vi "initialize.vi"(0 "MoAgSy_Engine":refnum<class "MoAgSy_Engine.lvclass">, 3 "initializationData":variant, 5 "error in (no error)":errorcluster, 7 "binaryString":string, 8 "I8 Array":i8[](array[numeric]), 9 "prependSize? (T)":bool, 11 "byteOrder (0:big-endian, network order)":T1(ring)) -> (14 "dup MoAgSy_Engine":refnum<class "MoAgSy_Engine.lvclass">, 17 "found?":bool, 19 "error out":errorcluster)   [LabVIEW 2009, in "MoAgSy.lvlib" / "MoAgSy_Engine.lvclass"]
doc: "This is a dynamic dispatch VI to be implemented by child classes to initialize their attributes.\n\n<B>Recommendation:</B> Use Variant for initialization data."
uses:
  MoAgSy_Engine.lvclass
  MoAgSy_AgentBase/MoAgSy_AgentBase.lvclass
  HGF_BaseClasses/HGF_Event/HGF_Event.lvclass
  HGF_BaseClasses/HGF_ThreadTask/HGF_ThreadTask.lvclass
  MoAgSy_Engine.lvclass/MoAgSy_Engine.ctl
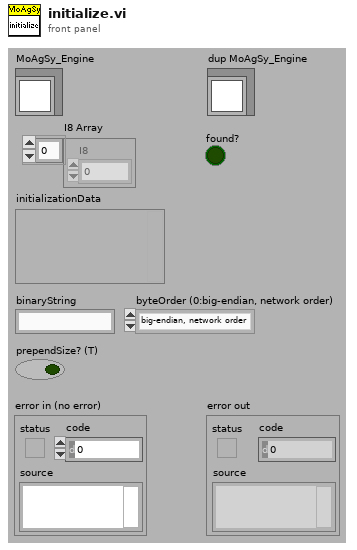
[diagram p1: front panel]
types:
  T1 = enum16{"big-endian, network order", "native, host order", "little-endian"}
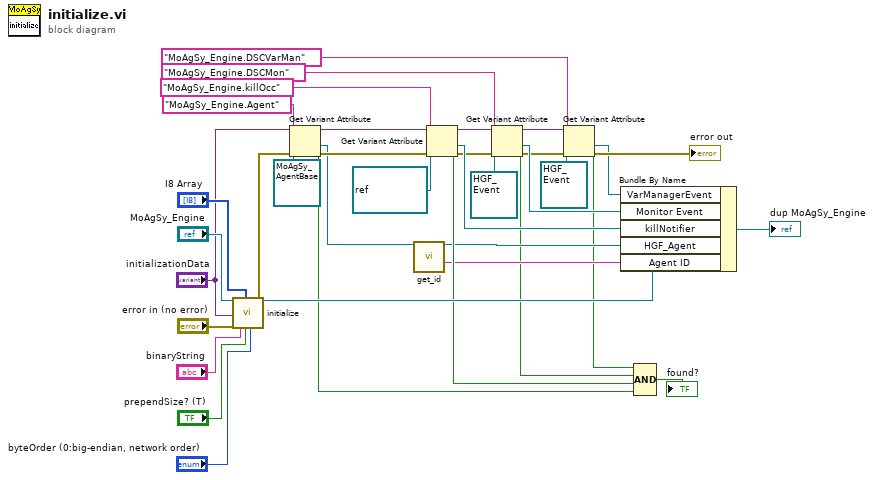
[diagram p0: block diagram]
diagram:
  n1 = call-parent "initialize.vi"("HGF_ThreadTask"="MoAgSy_Engine", "initializationData"="initializationData", "error in (no error)"="error in (no error)", "binaryString"="binaryString", "I8 Array"="I8 Array", "prependSize? (T)"="prependSize? (T)", "byteOrder (0:big-endian, network order)"="byteOrder (0:big-endian, network order)") -> ("dup HGF_ThreadTask"=w30:refnum<class "MoAgSy_Engine.lvclass">, "error out"=w23:errorcluster)  [unwired: 11 out]
  n2 = Get Variant Attribute(Variant="initializationData", name="MoAgSy_Engine.Agent", default value (empty Variant)=refnum<class "MoAgSy_AgentBase.lvclass"> refnum ("HGF_Agent"), error in=w23) -> (duplicate Variant=w27:variant, found=w21:bool, value=w18:refnum<class "MoAgSy_AgentBase.lvclass">, error out=w26:errorcluster)
  n3 = call "get_id.vi"("HGF_Agent in"=w18) -> ("HGF_Agent out"=w17:refnum<class "MoAgSy_AgentBase.lvclass">, "ID"=w16:string)  [unwired: 1 in, 16 out]
  n4 = Get Variant Attribute(Variant=w27, name="MoAgSy_Engine.killOcc", default value (empty Variant)=refnum<notifier> refnum ("killNotifier"), error in=w26) -> (duplicate Variant=w12:variant, found=w22:bool, value=w14:refnum<notifier>, error out=w13:errorcluster)
  n5 = Get Variant Attribute(Variant=w12, name="MoAgSy_Engine.DSCMon", default value (empty Variant)=refnum<class "HGF_Event.lvclass"> refnum ("HGF_Event (Monitor Event)"), error in=w13) -> (duplicate Variant=w6:variant, found=w10:bool, value=w9:refnum<class "HGF_Event.lvclass">, error out=w8:errorcluster)
  n6 = Get Variant Attribute(Variant=w6, name="MoAgSy_Engine.DSCVarMan", default value (empty Variant)=refnum<class "HGF_Event.lvclass"> refnum ("VarManagerEvent"), error in=w8) -> (found=w3:bool, value=w4:refnum<class "HGF_Event.lvclass">, error out=→"error out":errorcluster)  [unwired: 1 out]
  n7 = Bundle By Name(cluster=w30, "VarManagerEvent"=w4, "Monitor Event"=w9, "killNotifier"=w14, "HGF_Agent"=w17, "Agent ID"=w16) -> (→"dup MoAgSy_Engine":refnum<class "MoAgSy_Engine.lvclass">)
  n8 = Compound Arithmetic op=AND(w3, w10, w22, w21) -> (→"found?":bool)
